vi "LWXPS_PositionerPositionCompareSet.vi"(5 "LabVIEW error IN":errorcluster, 6 "XPS Reference IN":refnum<k24>, 7 "Position Step":dbl, 8 "Maximum Position":dbl, 9 "Minimum Position":dbl, 10 "Positioner Name":string) -> (0 "LabVIEW error OUT":errorcluster, 1 "XPS Error String":string, 2 "Returned error code":i32, 3 "XPS Reference OUT":refnum<k24>)   [LabVIEW 2014]
uses:
  D:/XPSQ8_LabView_Library/Development/Source/Dll/Newport.XPS.CommandInterface.dll
  Dll/Newport.XPS.CommandInterface.dll
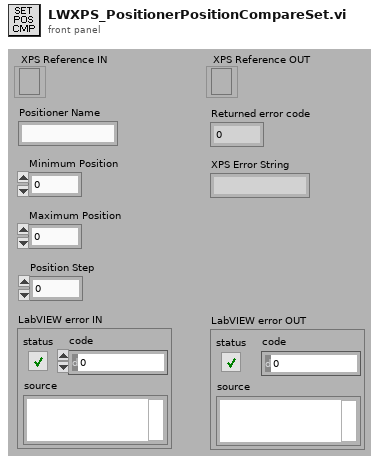
[diagram p1: front panel]
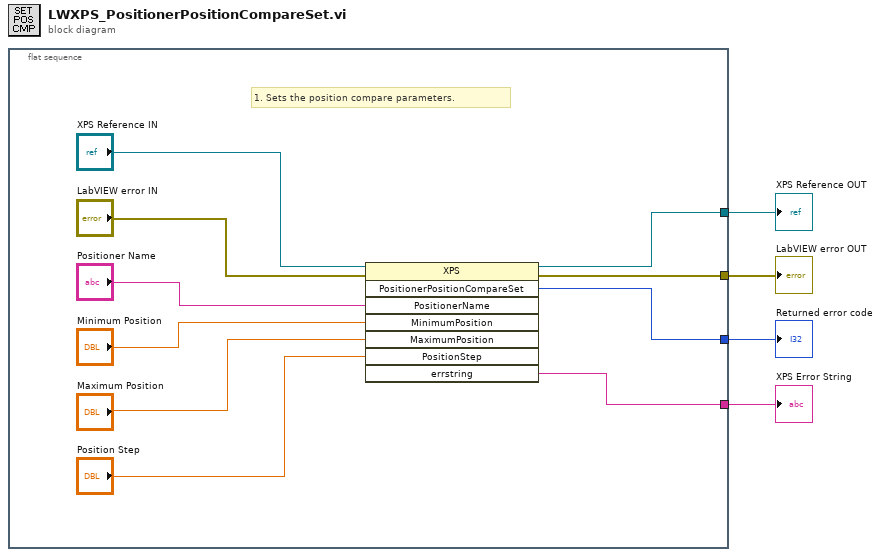
[diagram p0: block diagram]
diagram:
  n1 = flat-sequence {
    tunnel: [w10] -> w4
    tunnel: [w9] -> w3
    tunnel: [w11] -> w2
    tunnel: [w7] -> w1
    frame #0 {
      # "1. Sets the position compare parameters."
      n2 = invoke class="XPS" method="PositionerPositionCompareSet"(reference="XPS Reference IN", error in="LabVIEW error IN", "PositionerName"="Positioner Name", "MinimumPosition"="Minimum Position", "MaximumPosition"="Maximum Position", "PositionStep"="Position Step") -> (reference out=w10:refnum<k24>, error out=w9:errorcluster, "PositionerPositionCompareSet"=w11:i32, "errstring"=w7:string)  [unwired: 2 in, 4 out]
    }
  }
  "XPS Error String" <- w1
  "XPS Reference OUT" <- w4
  "LabVIEW error OUT" <- w3
  "Returned error code" <- w2
